vi "StateMachine_Temp_Hum_Sensor_SubVi_Acce.vi"() -> ()   [LabVIEW 2017]
uses:
  <vilib>/Instr/_visa.llb/VISA Configure Serial Port (Instr).vi
  <vilib>/Utility/file.llb/Write Delimited Spreadsheet (string).vi
  <vilib>/express/express shared/transition.llb/Dynamic To Waveform Array.vi
  <vilib>/express/express signal manip/GetorSetDDTAttributes/Set DDT Attributes/SetT0.vi
  <vilib>/express/express shared/transition.llb/Waveform Array To Dynamic.vi
  <vilib>/express/express signal manip/GetorSetDDTAttributes/Set DDT Attributes/Set DDT Properties.xnode
panel:
  in  "Tab Control":T1(tab)
  in  "Log File Path":path
  out "Humidity (%)":i32(graph)
  out "Heat Index (°C)":i32(graph)
  in  "Data Table":string[][](table)
  in  "stop 2":bool
  in  "VISA resource name":refnum<visa-resource-name>
  out "Temperature (°F)":i32(knob) scale=0.0..100.0
  out "Temperature (°C)":i32(knob) scale=0.0..100.0
  out "Temperature (°F)":i32(graph)
  out "Temperature (°C)":i32(graph)
  in  "Stop Test":bool
  in  "rate":dbl=1000.0
  in  "number of samples":i32=100
  in  "timeout (s)":dbl=10.0 format="%0.2f"
  out "Raw Accelerometer Voltage":dynamicdata(graph)
  out "Acceleration (m/s^2)":dynamicdata(graph)
  in  "Enable":bool=TRUE
  in  "Filename":path=path "C:/Users/Hp/Documents/GitCodes/LABVIEW PRACTICE 2024/test.lvm"
  out "Saving Data":bool
  out "Filename Out":path
  out "Filename Out":path
  out "Saving Data":bool
  in  "Filename 2":path=path "C:/Users/Hp/Documents/GitCodes/LABVIEW PRACTICE 2024/test.lvm" caption="Filename"
  in  "Enable 2":bool=TRUE caption="Enable"
  out "Accelerometer #1 Acceleration (m/s^2)":dynamicdata(graph)
  out "Raw Accelerometer Voltage 2":dynamicdata(graph) caption="Raw Accelerometer Voltage - Multiple Accelerometer"
  in  "timeout (s) 2":dbl=10.0 caption="timeout (s)" format="%0.2f"
  in  "number of samples 2":i32=100
  in  "rate 2":dbl=1000.0
  out "Accelerometer #2 Acceleration (m/s^2)":dynamicdata(graph)
  in  "Stop test":bool
  in  "Error In 2":errorcluster
  out "Heat Index (°F)":string
  out "Numeric 3":i32
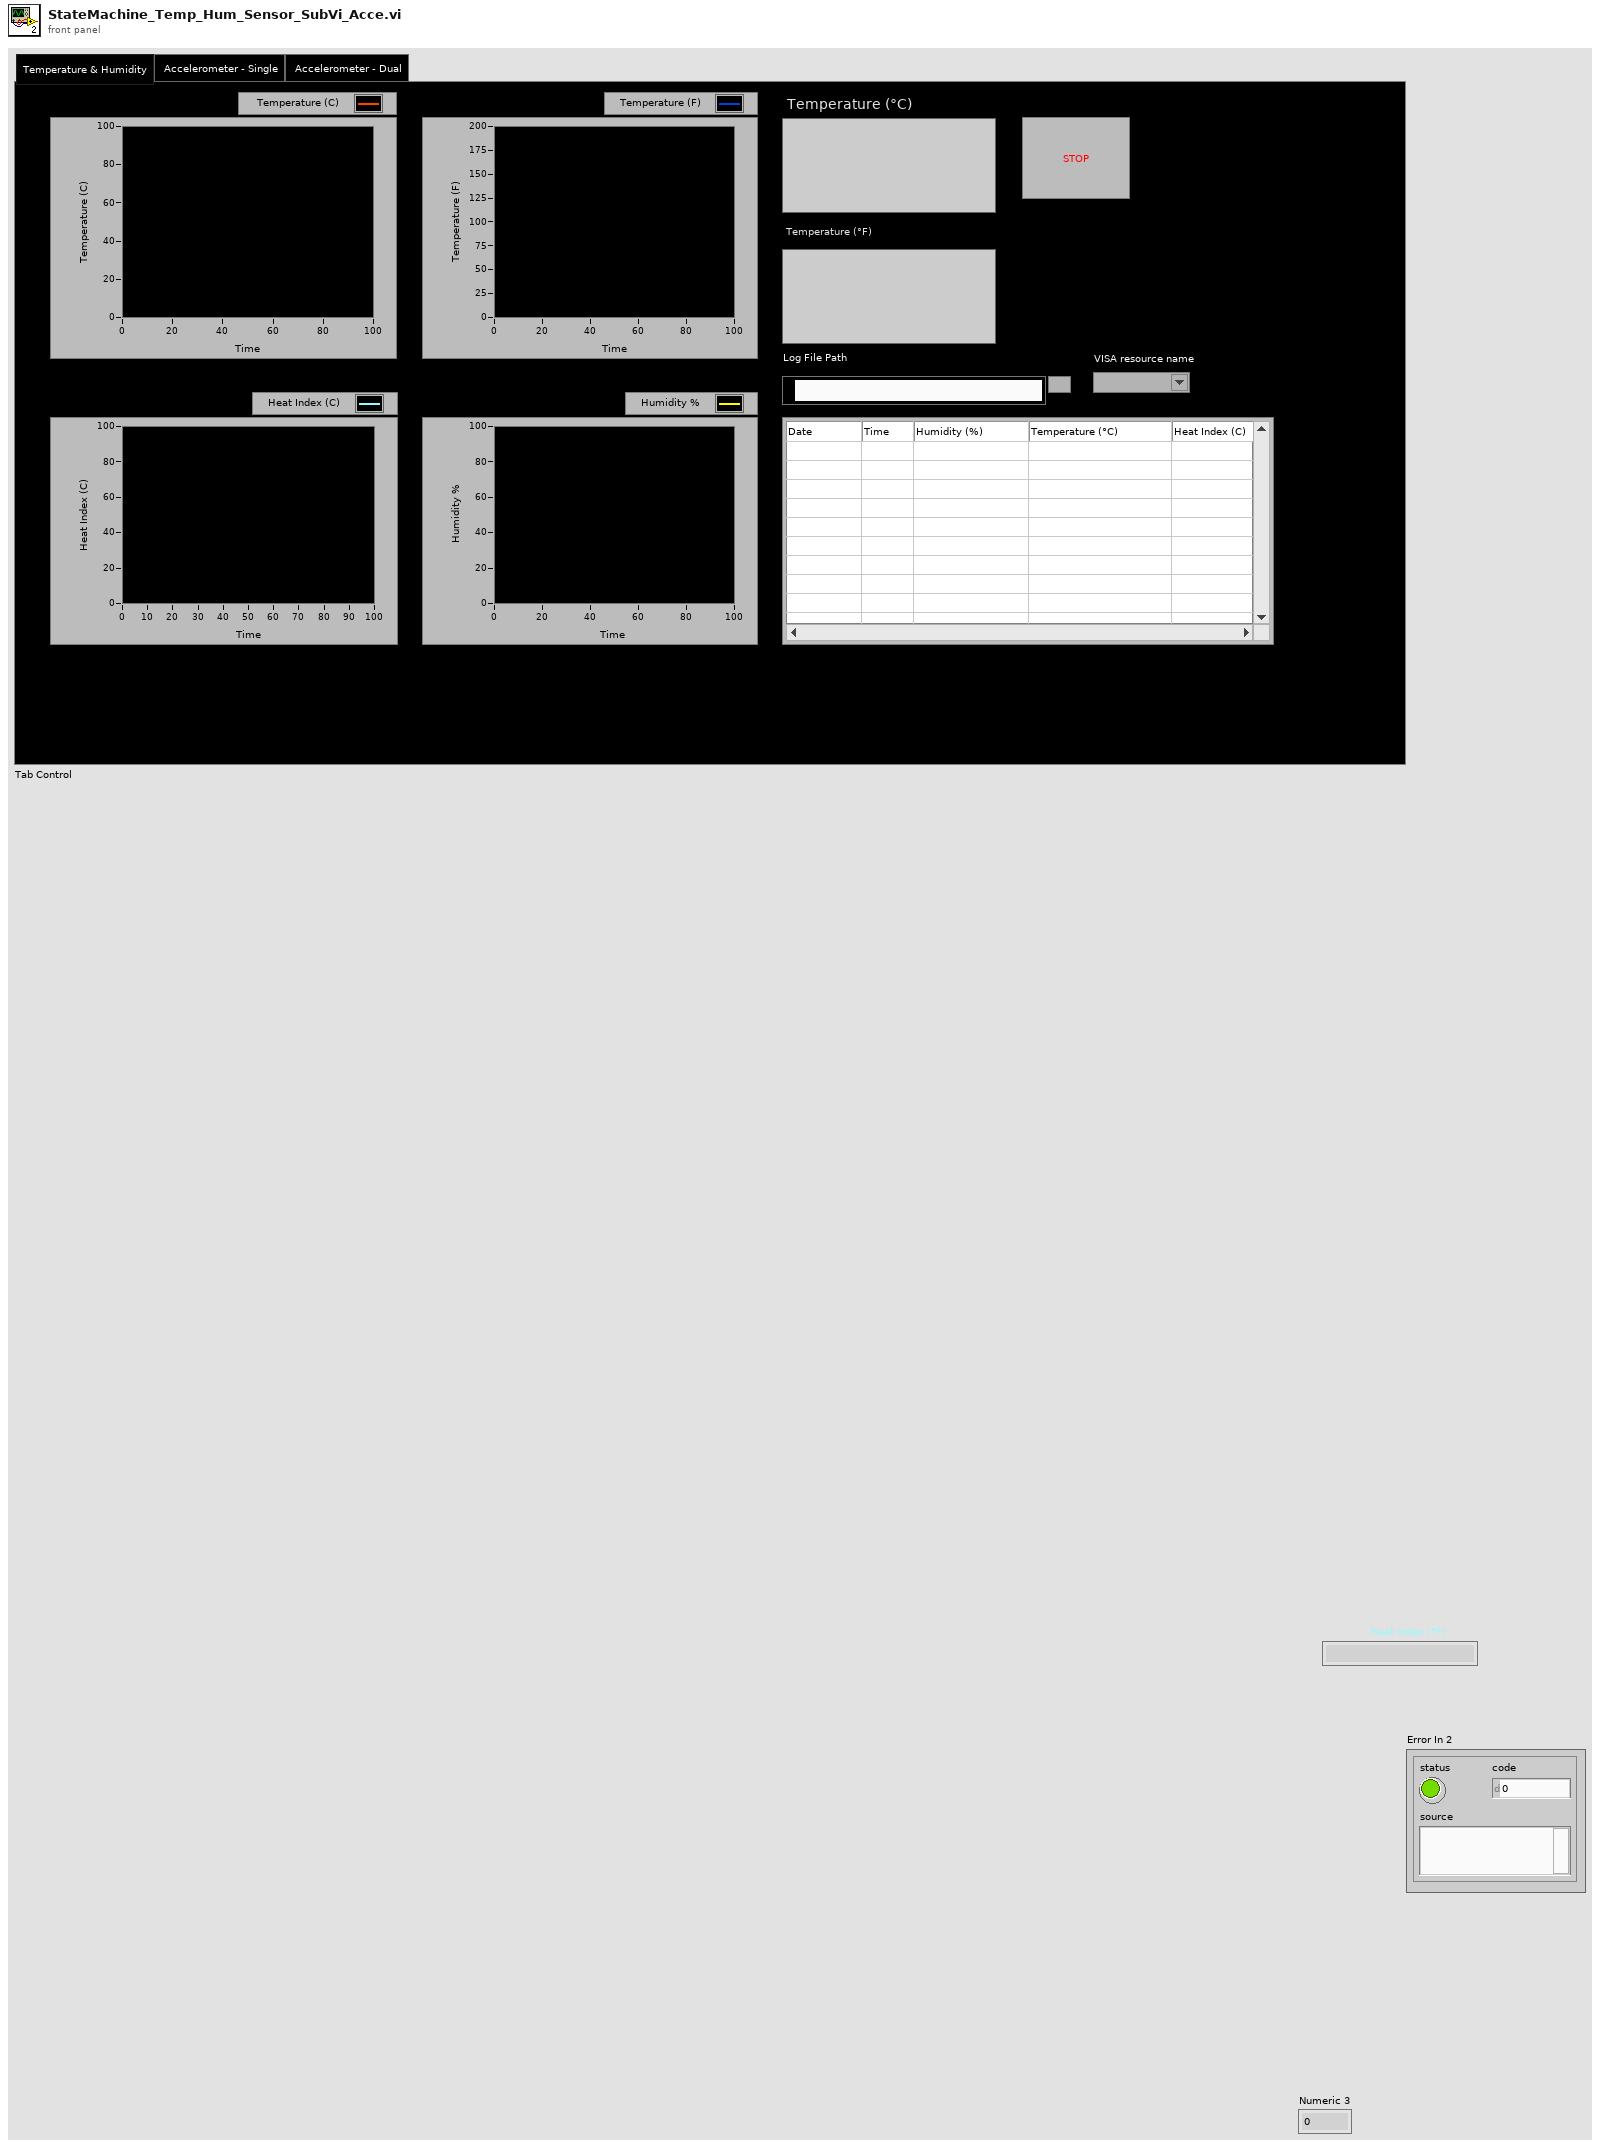
[diagram p1: front panel]
types:
  T1 = enum32{"Temperature & Humidity", " Accelerometer - Single", " Accelerometer - Dual"}
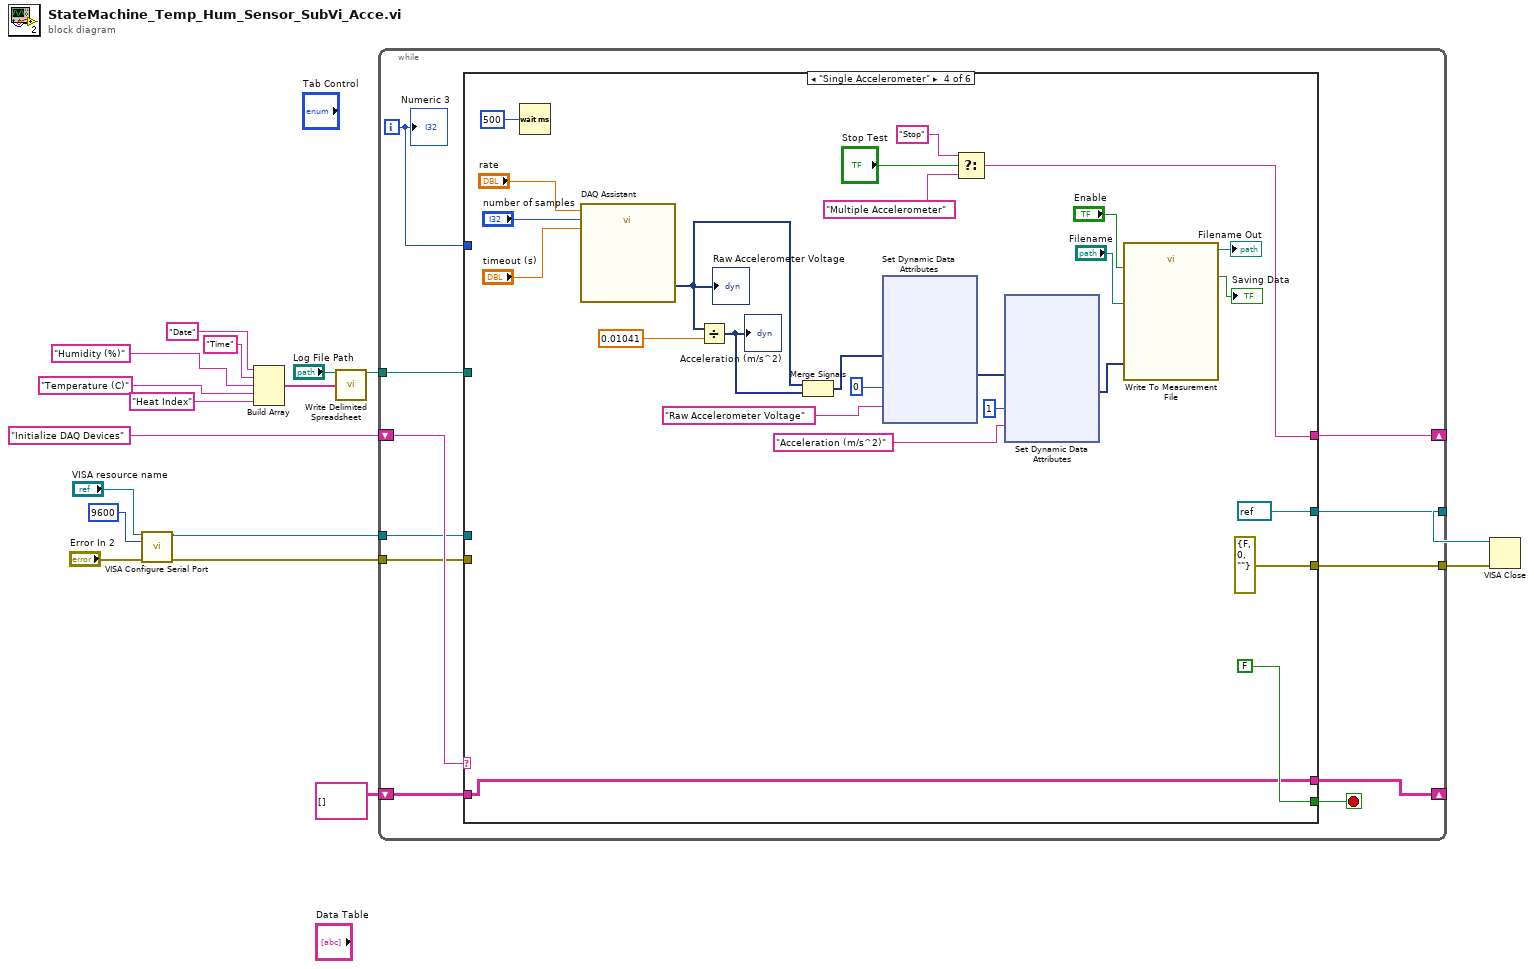
[diagram p0: block diagram]
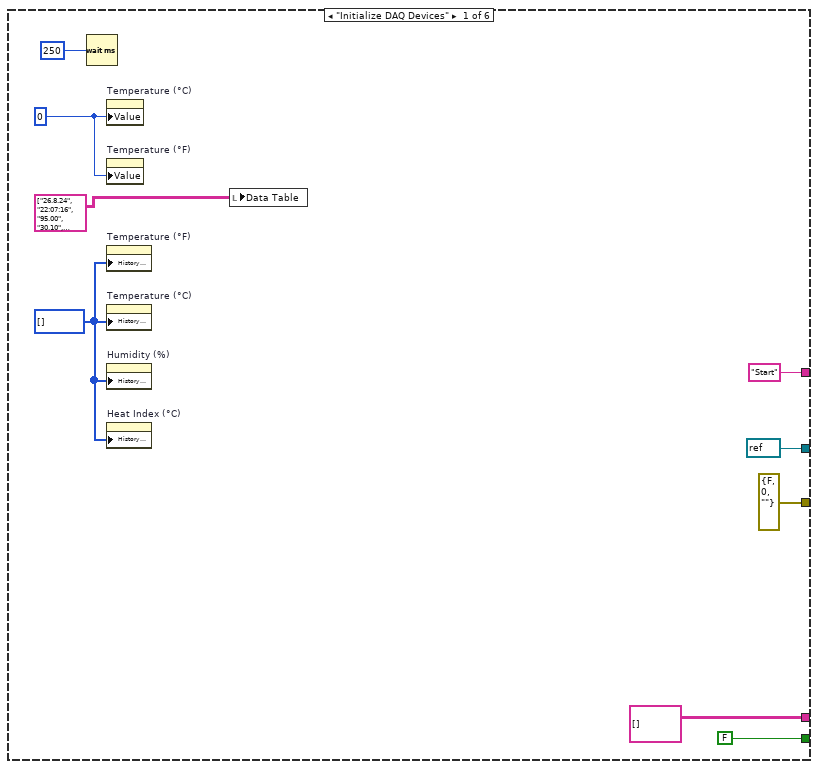
[diagram p2: hidden frame]
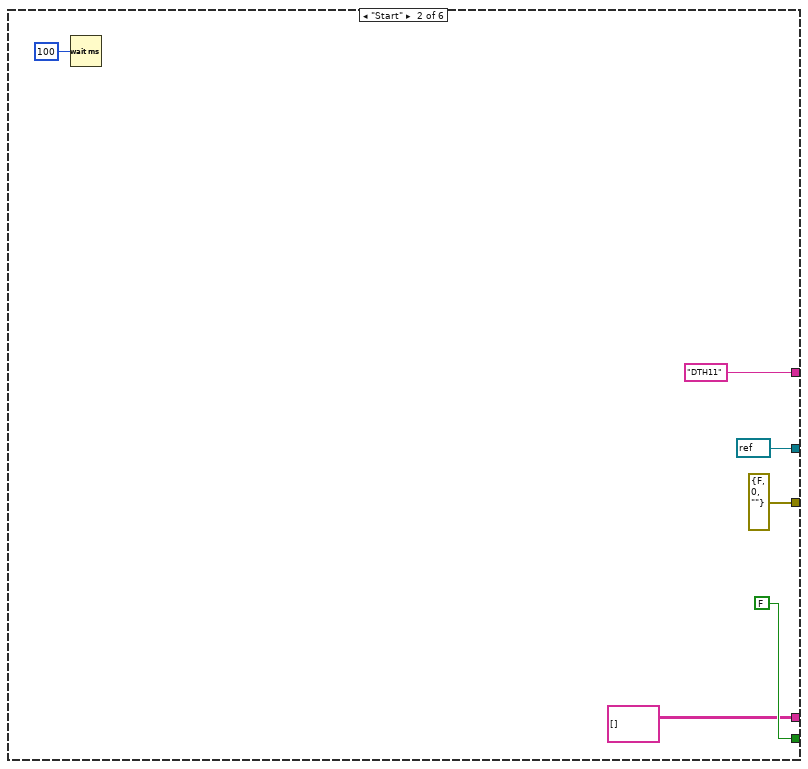
[diagram p3: hidden frame]
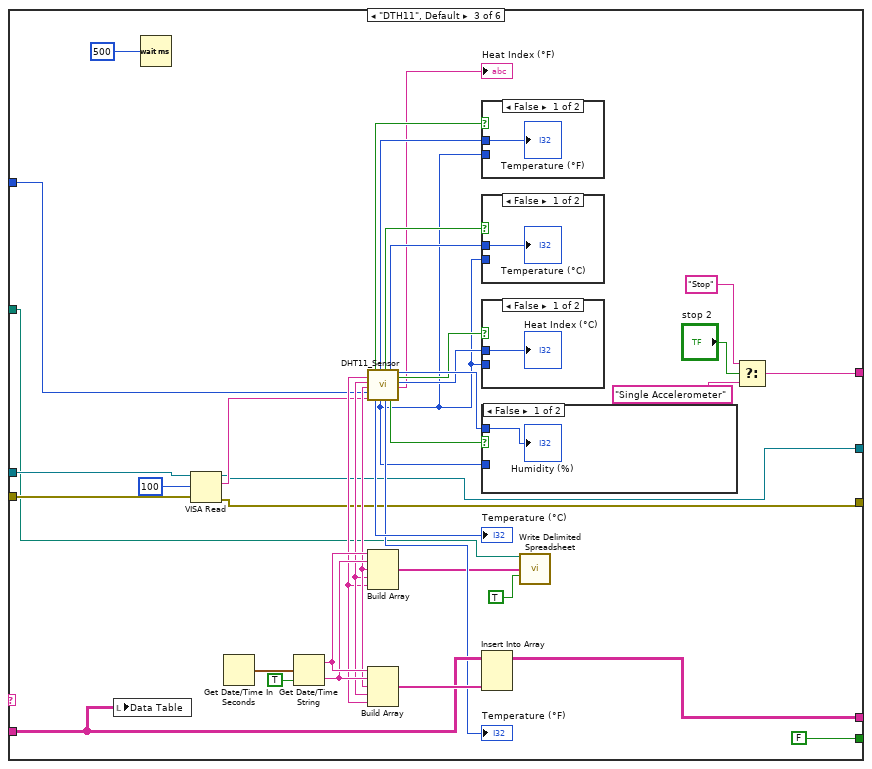
[diagram p4: hidden frame]
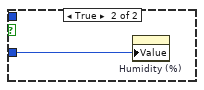
[diagram p5: hidden frame]
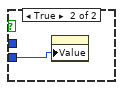
[diagram p6: hidden frame]
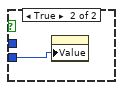
[diagram p7: hidden frame]
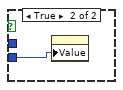
[diagram p8: hidden frame]
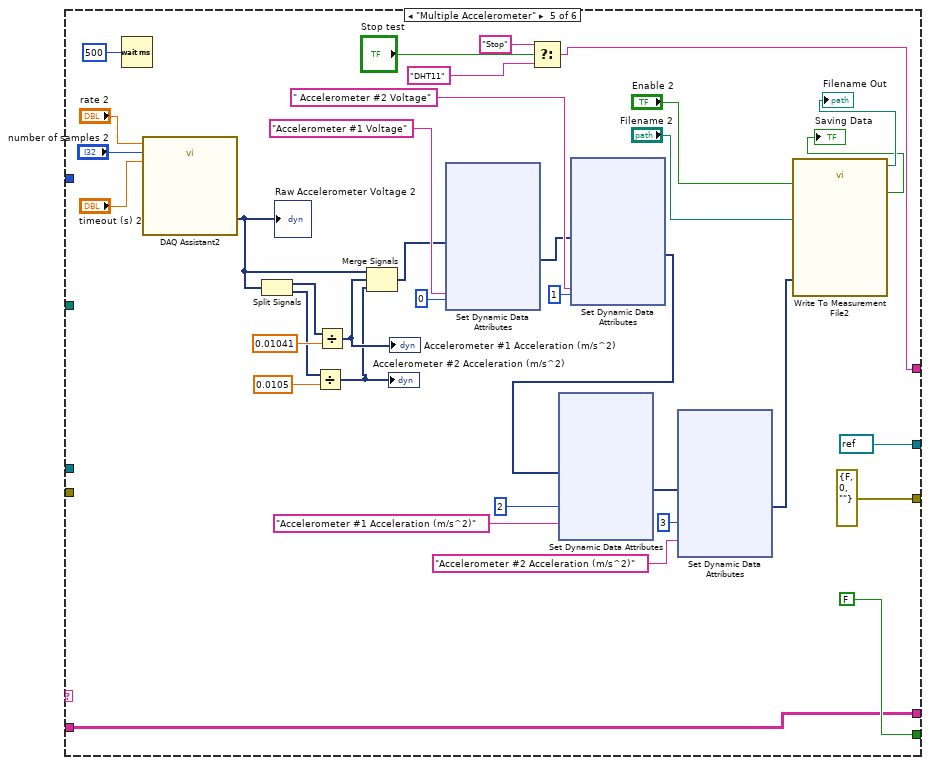
[diagram p9: hidden frame]
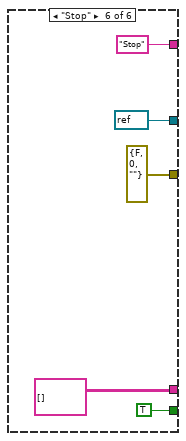
[diagram p10: hidden frame]
diagram:
  n1 = call-poly "VISA Configure Serial Port"("VISA resource name"="VISA resource name", "baud rate (9600)"=u32 9600, "error in (no error)"="Error In 2") -> ("VISA resource name out"=w10:refnum<visa-resource-name>, "error out"=w11:errorcluster)  [unwired: 11 in]
  n2 = Build Array("Date" ("regular expression"), "Time" ("regular expression"), "Humidity (%)" ("regular expression"), "Temperature (C)" ("regular expression"), "Heat Index" ("element")) -> (w5:string[])
  n3 = call-poly <vilib>:"Write Delimited Spreadsheet.vi"("file path (dialog if empty)"="Log File Path", "1D data"=w5) -> ("new file path (Not A Path if cancelled)"=w3:path)  [unwired: 12 in, 1 out]
  n4 = while {
    shift-right: [w28] -> _
    shift-left: "Initialize DAQ Devices" -> [w27]
    tunnel: [w19] -> w16
    tunnel: [w20] -> w15
    shift-right: [w24] -> _
    shift-left: string[][] [] -> [w25]
    tunnel: w10 -> [w22]
    tunnel: w11 -> [w21]
    tunnel: w3 -> [w18]
    i -> [w23]
    stop <- w26 stop-if-true
    n5 = case shown="\"Single Accelerometer\"" w27 {
      tunnel: ["Start" "DTH11" w70 w92 w144 "Stop"] -> w28
      tunnel: w25 -> [_ _ w72 w91 w143 _]
      tunnel: [errorcluster {"status"=FALSE, "code"=0, "source"=""} ("error out") errorcluster {"status"=FALSE, "code"=0, "source"=""} ("error out") w50 errorcluster {"status"=FALSE, "code"=0, "source"=""} ("error out") errorcluster {"status"=FALSE, "code"=0, "source"=""} ("error out") errorcluster {"status"=FALSE, "code"=0, "source"=""} ("error out")] -> w19
      tunnel: [string[][] [] string[][] [] w71 w91 w143 string[][] []] -> w24
      tunnel: [FALSE FALSE FALSE FALSE FALSE TRUE] -> w26
      tunnel: [refnum<visa-resource-name> refnum ("VISA resource name out") refnum<visa-resource-name> refnum ("VISA resource name out") w47 refnum<visa-resource-name> refnum ("VISA resource name out") refnum<visa-resource-name> refnum ("VISA resource name out") refnum<visa-resource-name> refnum ("VISA resource name out")] -> w20
      tunnel: w23 -> [_ _ w53 _ _ _]
      tunnel: w22 -> [_ _ w51 _ _ _]
      tunnel: w21 -> [_ _ w49 _ _ _]
      tunnel: w18 -> [_ _ w44 _ _ _]
      frame "Initialize DAQ Devices" {
        w30 = 0 ("Temperature (°F) 2")
        w32 = i32[] [] ("History Data")
        n6 = Wait (ms)(milliseconds to wait=u32 250) -> ()  [unwired: 1 out]
        n7 = property on="Temperature (°C)" class="Knob (strict)"("Value"=w30) -> ()  [unwired: 2 in, 2 out]
        n8 = property on="Temperature (°F)" class="Knob (strict)"("Value"=w30) -> ()  [unwired: 2 in, 2 out]
        n9 = property on="Temperature (°F)" class="WFChart (strict)"("History Data"=w32) -> ()  [unwired: 2 in, 2 out]
        n10 = property on="Temperature (°C)" class="WFChart (strict)"("History Data"=w32) -> ()  [unwired: 2 in, 2 out]
        n11 = property on="Humidity (%)" class="WFChart (strict)"("History Data"=w32) -> ()  [unwired: 2 in, 2 out]
        n12 = property on="Heat Index (°C)" class="WFChart (strict)"("History Data"=w32) -> ()  [unwired: 2 in, 2 out]
        n13 = local write "Data Table"(string[][] [["26.8.24", "22:07:16", "95.00", "30.10", "42.92"], ["26.8.24", "22:07:17", "95.00", "30.10", "42.92"], ["26.8.24", "22:07:18", "95.00", "30.10", "42.92"], ["26.8.24", "22:07:19", "95.00", "30.10", "42.92"], ["26.8.24", "22:07:20", "93.00", "30.10", "42.20"], ["26.8.24", "22:07:21", "92.00", "30.10", "41.84"], ["26.8.24", "22:07:22", "90.00", "30.10", "41.15"], ["26.8.24", "22:07:23", "90.00", "30.10", "41.15"], ["26.8.24", "22:07:24", "89.00", "30.10", "40.80"], ["26.8.24", "22:07:25", "88.00", "30.10", "40.47"], ["26.8.24", "22:07:26", "88.00", "30.10", "40.47"], ["26.8.24", "22:07:27", "87.00", "30.10", "40.14"], ["26.8.24", "22:07:28", "86.00", "30.10", "39.81"], ["26.8.24", "22:07:29", "86.00", "30.00", "39.46"], ["26.8.24", "22:07:30", "86.00", "30.00", "39.46"], ["26.8.24", "22:07:31", "85.00", "30.00", "39.14"], ["26.8.24", "22:07:32", "85.00", "30.00", "39.14"], ["26.8.24", "22:07:33", "85.00", "29.90", "38.80"], ["26.8.24", "22:07:34", "85.00", "30.00", "39.14"], ["26.8.24", "22:07:35", "84.00", "30.00", "38.84"], ["26.8.24", "22:07:36", "84.00", "29.90", "38.50"], ["26.8.24", "22:07:37", "84.00", "29.90", "38.50"], ["26.8.24", "22:07:38", "84.00", "29.90", "38.50"], ["26.8.24", "22:07:39", "84.00", "29.90", "38.50"], ["26.8.24", "22:07:40", "84.00", "29.90", "38.50"], ["26.8.24", "22:07:41", "84.00", "29.80", "38.17"], ["26.8.24", "22:07:42", "83.00", "29.80", "37.89"], ["26.8.24", "22:07:43", "83.00", "29.80", "37.89"], ["26.8.24", "22:07:44", "84.00", "29.80", "38.17"], ["26.8.24", "22:07:45", "84.00", "29.70", "37.85"], ["26.8.24", "22:07:46", "84.00", "29.70", "37.85"], ["26.8.24", "22:07:47", "84.00", "29.70", "37.85"], ["26.8.24", "22:07:48", "83.00", "29.70", "37.57"], ["26.8.24", "22:07:49", "83.00", "29.70", "37.57"], ["26.8.24", "22:07:50", "83.00", "29.70", "37.57"], ["26.8.24", "22:07:51", "83.00", "29.70", "37.57"], ["26.8.24", "22:07:52", "83.00", "29.70", "37.57"], ["26.8.24", "22:07:53", "83.00", "29.70", "37.57"], ["26.8.24", "22:07:54", "83.00", "29.70", "37.57"], ["26.8.24", "22:07:55", "84.00", "29.70", "37.85"], ["26.8.24", "22:07:56", "83.00", "29.70", "37.57"], ["26.8.24", "22:07:57", "83.00", "29.60", "37.25"], ["26.8.24", "22:07:58", "83.00", "29.60", "37.25"], ["26.8.24", "22:07:59", "83.00", "29.60", "37.25"], ["26.8.24", "22:08:00", "83.00", "29.60", "37.25"], ["26.8.24", "22:08:01", "83.00", "29.60", "37.25"], ["26.8.24", "22:08:02", "83.00", "29.60", "37.25"], ["26.8.24", "22:08:03", "84.00", "29.60", "37.52"], ["26.8.24", "22:08:04", "84.00", "29.60", "37.52"], ["26.8.24", "22:08:05", "84.00", "29.60", "37.52"], ["26.8.24", "22:08:06", "84.00", "29.60", "37.52"], ["26.8.24", "22:08:07", "83.00", "29.60", "37.25"], ["26.8.24", "22:08:08", "83.00", "29.60", "37.25"], ["26.8.24", "22:08:09", "83.00", "29.60", "37.25"], ["26.8.24", "22:08:10", "83.00", "29.60", "37.25"], ["26.8.24", "22:08:11", "83.00", "29.50", "36.94"], ["26.8.24", "22:08:12", "83.00", "29.50", "36.94"], ["26.8.24", "22:08:13", "83.00", "29.50", "36.94"], ["26.8.24", "22:08:14", "83.00", "29.50", "36.94"], ["26.8.24", "22:08:15", "83.00", "29.50", "36.94"], ["26.8.24", "22:08:16", "83.00", "29.50", "36.94"], ["26.8.24", "22:08:17", "83.00", "29.50", "36.94"], ["26.8.24", "22:08:18", "83.00", "29.50", "36.94"], ["26.8.24", "22:08:19", "83.00", "29.50", "36.94"], ["26.8.24", "22:08:20", "83.00", "29.50", "36.94"], ["26.8.24", "22:08:21", "83.00", "29.50", "36.94"], ["26.8.24", "22:08:22", "83.00", "29.50", "36.94"], ["26.8.24", "22:08:23", "83.00", "29.50", "36.94"], ["26.8.24", "22:08:24", "83.00", "29.50", "36.94"], ["26.8.24", "22:08:25", "83.00", "29.40", "36.62"], ["26.8.24", "22:08:26", "83.00", "29.50", "36.94"], ["26.8.24", "22:08:27", "Failed to read from DHT sensor!\r\n", "", ""], ["26.8.24", "22:08:28", "95.00", "29.40", "40.17"], ["26.8.24", "22:08:29", "95.00", "29.50", "40.55"], ["26.8.24", "22:08:30", "95.00", "29.50", "40.55"], ["26.8.24", "22:08:31", "95.00", "29.60", "40.94"], ["26.8.24", "22:08:32", "95.00", "29.70", "41.33"]] ("Data Table")) -> ()
      }
      frame "Start" {
        n14 = Wait (ms)(milliseconds to wait=u32 100) -> ()  [unwired: 1 out]
      }
      frame "DTH11", Default {
        n15 = local write "Data Table"(w72) -> ()
        n16 = Wait (ms)(milliseconds to wait=u32 500) -> ()  [unwired: 1 out]
        n17 = VISA Read(VISA resource name=w51, byte count=u32 100, error in (no error)=w49) -> (VISA resource name out=w47:refnum<visa-resource-name>, read buffer=w48:string, error out=w50:errorcluster)  [unwired: 1 out]
        n18 = Get Date/Time In Seconds() -> (seconds since 1Jan1904=w73:timestamp)
        n19 = Get Date/Time String(seconds (now)=w73, want seconds? (F)=TRUE) -> (date string=w75:string, time string=w74:string)  [unwired: 1 in]
        n20 = call "DHT11_Sensor.vi"("Iteration Terminal"=w53, "Serial String"=w48) -> ("Heat Index (°C) 2"=w54:string, "Temperature (°C) 3"=w55:string, "Humidity (%) 2"=w56:string, "Temperature (F)"=w68:bool, "T emperature (F)"=→"Temperature (°C)":i32, "T (F) Plot False Case"=w67:i32, "T (F) True Case"=w58:i32, "Temperature (C)"=w65:bool, "Temperature (°C)"=→"Temperature (°F)":i32, "T (C) Plot False Case"=w64:i32, "Humidity"=w62:bool, "Humidity %"=w61:i32, "Heat Index"=w60:bool, "Heat Index (C)"=w59:i32, "Heat Index (F)"=→"Heat Index (°F)":string)  [unwired: 3 in]
        n21 = Build Array "Build Array"(w75, w74, w56, w55, w54) -> (w45:string[])
        n22 = Build Array "Build Array"(w75, w74, w56, w55, w54) -> (w77:string[])
        n23 = case shown="False" w68 {
          tunnel: w67 -> [w88 _]
          tunnel: w58 -> [_ w89]
          frame False {
            "Temperature (°F)" <- w88
          }
          frame True {
            n24 = property on="Temperature (°F)" class="WFChart (strict)"("Value"=w89) -> ()  [unwired: 2 in, 2 out]
          }
        }
        n25 = case shown="False" w65 {
          tunnel: w64 -> [w84 _]
          tunnel: w58 -> [_ w85]
          frame False {
            "Temperature (°C)" <- w84
          }
          frame True {
            n26 = property on="Temperature (°C)" class="WFChart (strict)"("Value"=w85) -> ()  [unwired: 2 in, 2 out]
          }
        }
        n27 = case shown="False" w60 {
          tunnel: w59 -> [w86 _]
          tunnel: w58 -> [_ w87]
          frame False {
            "Heat Index (°C)" <- w86
          }
          frame True {
            n28 = property on="Heat Index (°C)" class="WFChart (strict)"("Value"=w87) -> ()  [unwired: 2 in, 2 out]
          }
        }
        n29 = case shown="False" w62 {
          tunnel: w61 -> [w82 _]
          tunnel: w58 -> [_ w83]
          frame False {
            "Humidity (%)" <- w82
          }
          frame True {
            n30 = property on="Humidity (%)" class="WFChart (strict)"("Value"=w83) -> ()  [unwired: 2 in, 2 out]
          }
        }
        n31 = Insert Into Array "Insert Into Array"(array=w72, new element=w77) -> (w71:string[][])  [unwired: 2 in]
        n32 = call-poly <vilib>:"Write Delimited Spreadsheet.vi"("file path (dialog if empty)"=w44, "1D data"=w45, "append to file? (new file:F)"=TRUE) -> ()  [unwired: 11 in, 2 out]
        n33 = Select(t="Stop", s="stop 2", f="Single Accelerometer") -> (s? t:f=w70:string)
      }
      frame "Single Accelerometer" {
        n34 = Wait (ms)(milliseconds to wait=u32 500) -> ()  [unwired: 1 out]
        n35 = call "DAQ Assistant"("rate"="rate", "number of samples"="number of samples", "timeout (s)"="timeout (s)") -> ("data"=w107:dynamicdata)  [unwired: 14 in, 2 out]
        "Raw Accelerometer Voltage" <- w107
        n36 = Divide(x=w107, y=0.01041) -> (x/y=w106:dynamicdata)
        "Acceleration (m/s^2)" <- w106
        n37 = Merge Signals "Merge Signals"(w107, w106) -> (w103:dynamicdata)
        n38 = xnode "Set Dynamic Data Attributes"("Signals In"=w103, "Signal Index"=0, "Signal Name"="Raw Accelerometer Voltage") -> ("Signals Out"=w100:dynamicdata)  [unwired: 1 in, 1 out]
        n39 = Select(t="Stop", s="Stop Test", f="Multiple Accelerometer") -> (s? t:f=w92:string)
        n40 = xnode "Set Dynamic Data Attributes"("Signals In"=w100, "Signal Index"=1, "Signal Name"="Acceleration (m/s^2)") -> ("Signals Out"=w95:dynamicdata)  [unwired: 1 in, 1 out]
        n41 = call "Write To Measurement File"("Signals"=w95, "Enable"="Enable", "Filename"="Filename") -> ("Filename Out"=→"Filename Out":path, "Saving Data"=→"Saving Data":bool)  [unwired: 14 in, 1 out]
      }
      frame "Multiple Accelerometer" {
        n42 = Wait (ms)(milliseconds to wait=u32 500) -> ()  [unwired: 1 out]
        n43 = call "DAQ Assistant2"("rate"="rate 2", "number of samples"="number of samples 2", "timeout (s)"="timeout (s) 2") -> ("data"=w160:dynamicdata)  [unwired: 14 in, 2 out]
        "Raw Accelerometer Voltage 2" <- w160
        n44 = Split Signals(w160) -> (w157:dynamicdata, w155:dynamicdata)  [unwired: 2 in]
        n45 = Divide(x=w155, y=0.0105) -> (x/y=w154:dynamicdata)
        "Accelerometer #2 Acceleration (m/s^2)" <- w154
        n46 = Divide(x=w157, y=0.01041) -> (x/y=w156:dynamicdata)
        "Accelerometer #1 Acceleration (m/s^2)" <- w156
        n47 = Merge Signals(w160, w156, w154) -> (w168:dynamicdata)
        n48 = xnode "Set Dynamic Data Attributes"("Signals In"=w168, "Signal Index"=0, "Signal Name"="Accelerometer #1 Voltage") -> ("Signals Out"=w165:dynamicdata)  [unwired: 1 in, 1 out]
        n49 = Select(t="Stop", s="Stop test", f="DHT11") -> (s? t:f=w144:string)
        n50 = xnode "Set Dynamic Data Attributes"("Signals In"=w165, "Signal Index"=1, "Signal Name"=" Accelerometer #2 Voltage") -> ("Signals Out"=w148:dynamicdata)  [unwired: 1 in, 1 out]
        n51 = xnode "Set Dynamic Data Attributes"("Signals In"=w148, "Signal Index"=2, "Signal Name"="Accelerometer #1 Acceleration (m/s^2)") -> ("Signals Out"=w153:dynamicdata)  [unwired: 1 in, 1 out]
        n52 = xnode "Set Dynamic Data Attributes"("Signals In"=w153, "Signal Index"=3, "Signal Name"="Accelerometer #2 Acceleration (m/s^2)") -> ("Signals Out"=w147:dynamicdata)  [unwired: 1 in, 1 out]
        n53 = call "Write To Measurement File2"("Signals"=w147, "Enable"="Enable 2", "Filename"="Filename 2") -> ("Filename Out"=→"Filename Out":path, "Saving Data"=→"Saving Data":bool)  [unwired: 14 in, 1 out]
      }
      frame "Stop" {
      }
    }
    "Numeric 3" <- w23
  }
  n54 = VISA Close(VISA resource name=w15, error in (no error)=w16) -> ()  [unwired: 1 out]
